vi "Count Coins.vi"() -> ()   [LabVIEW 2022 SP3]
uses:
  Features.ctl
  <vilib>/userdefined/High Color/IMAQdx.ctl
  <vilib>/vision/driver/NI_Vision_Acquisition_Software.lvlib
panel:
  out "Features":cluster{"x":i32, "y":i32, "diameter":i32}[](array[cluster])
  out "Image":T1(plugin-control)
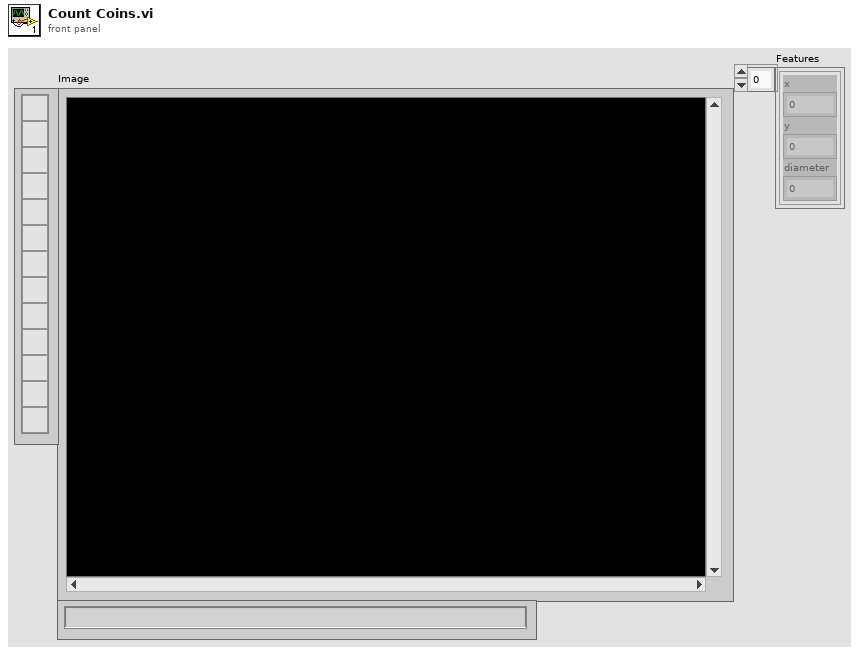
[diagram p1: front panel]
types:
  T1 = typedef "IMAQ Image.ctl" = refnum<image>
  T2 = typedef "Features.ctl" = cluster{"x":i32, "y":i32, "diameter":i32}
  T3 = typedef "IMAQdx.ctl" = refnum<k21>
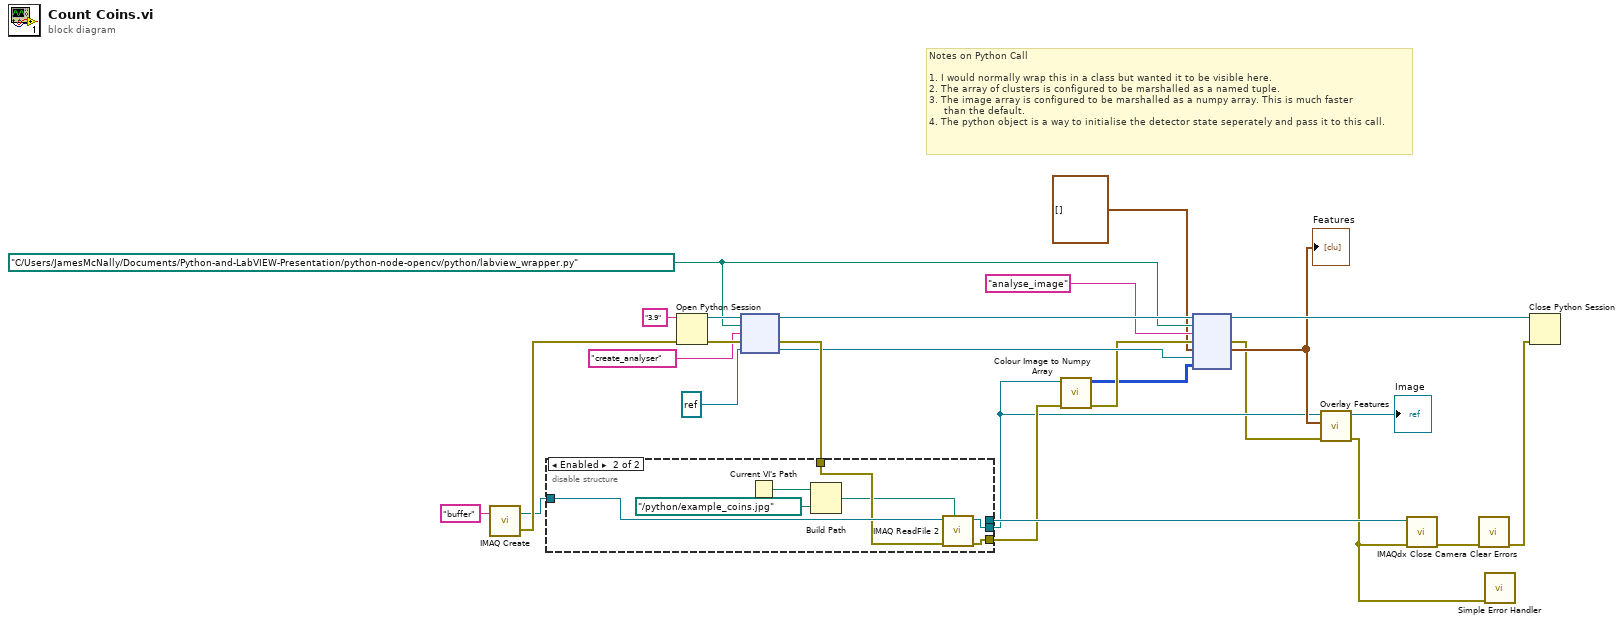
[diagram p0: block diagram]
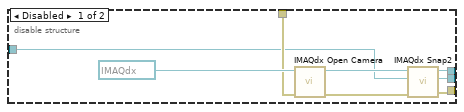
[diagram p2: hidden frame]
diagram:
  w16 = path "C:/Users/JamesMcNally/Documents/Python-and-LabVIEW-Presentation/python-node-opencv/python/labview_wrapper.py" ("module path")
  # "Notes on Python Call\n\n1. I would normally wrap this in a class but wanted it to be visible here.\n2. The array of clusters is configured to be marshalled as a named tuple.\n3. The image array is configured to be marshalled as a numpy array. This is much faster\n     than the default.\n4. The python object is a way to initialise the detector state seperately and pass it to this call."
  n1 = call "IMAQ Create"("Image Name"="buffer") -> ("New Image"=w8:T1, "error out"=w9:errorcluster)  [unwired: 4 in]
  n2 = Open Python Session(python version="3.9" ("Python version"), 3:w9) -> (session out=w22:refnum<k35>, error out=w21:errorcluster)  [unwired: 1 in]
  n3 = node(w22, w16, "create_analyser" ("function name"), w21, refnum<k38> refnum ("Python Object Refnum")) -> (w18:refnum<k35>, w20:errorcluster, w14:refnum<k38>)  [unwired: 2 out]
  n4 = disable-structure shown="Enabled" {
    disable-tunnel: [w32 _] -> w23
    disable-tunnel: w20 -> [w31 w38]
    disable-tunnel: [w30 w41] -> w5
    disable-tunnel: [w29 w40] -> w13
    disable-tunnel: w8 -> [w27 w39]
    frame Disabled {
      n5 = call <vilib>:"IMAQdx Open Camera.vi"("error in"=w31, "Session In"=T3 "cam0") -> ("error out"=w28:errorcluster, "Session Out"=w34:T3)  [unwired: 8 in]
      n6 = call <vilib>:"IMAQdx Snap2.vi"("error in"=w28, "Image In"=w27, "Session In"=w34) -> ("error out"=w29:errorcluster, "Image Out"=w30:T1, "Session Out"=w32:T3)  [unwired: 6 in]
    }
    frame Enabled {
      n7 = Current VI's Path() -> (path=w37:path)
      n8 = Build Path(base path=w37, name or relative path=path "../python/example_coins.jpg") -> (appended path=w35:path)
      n9 = call "IMAQ ReadFile 2"("File Path"=w35, "error in (no error)"=w38, "Image"=w39) -> ("error out"=w40:errorcluster, "Image Out"=w41:T1)  [unwired: 4 in, 3 out]
    }
  }
  n10 = call "Colour Image to Numpy Array.vi"("error in (no error)"=w13, "Refnum in"=w5) -> ("error out"=w12:errorcluster, "Array"=w3:u8[][][])  [unwired: 8 in]
  n11 = node(w18, w16, "analyse_image" ("function name"), w12, T2[] [], w14, w3) -> (w17:refnum<k35>, w2:errorcluster, w6:T2[])  [unwired: 2 in, 2 out]
  "Features" <- w6
  n12 = call "Overlay Features.vi"("error in (no error)"=w2, "Features"=w6, "Refnum in"=w5) -> ("Error Out"=w1:errorcluster, "Refnum out"=→"Image":T1)  [unwired: 7 in]
  n13 = call <vilib>:"IMAQdx Close Camera.vi"("error in"=w1, "Session In"=w23) -> ("error out"=w24:errorcluster)  [unwired: 9 in]
  n14 = call <vilib>:"Clear Errors.vi"("error in (no error)"=w24) -> ("error out"=w7:errorcluster)  [unwired: 5 in, 1 out]
  n15 = call <vilib>:"Simple Error Handler.vi"("error in (no error)"=w1) -> ()  [unwired: 4 in, 5 out]
  n16 = Close Python Session(session in=w17, error in=w7) -> ()  [unwired: 1 out]
